vi "Stop Module Event.vi"(8 "error in (no error)":errorcluster, 11 "Action":enum16{"Create", "Get", "Destroy"}(ring)=enum."Destroy") -> (0 "error out":errorcluster, 3 "Stop Module":refnum<user-event>)   [LabVIEW 2018]
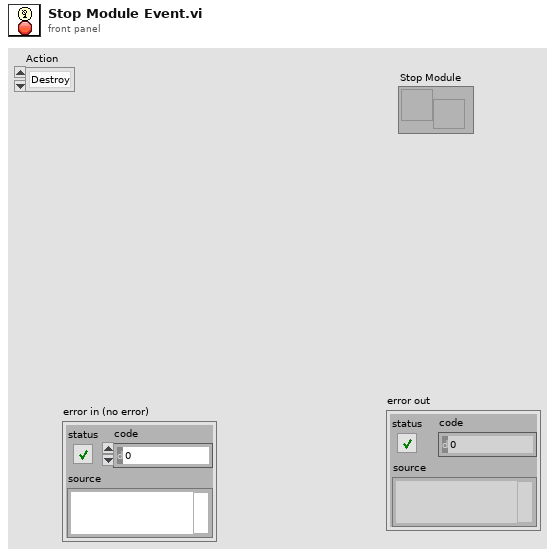
[diagram p1: front panel]
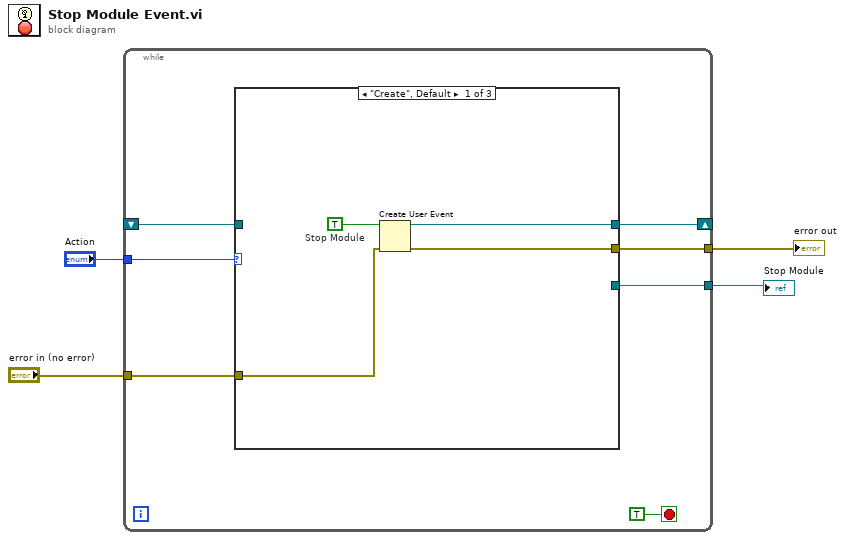
[diagram p0: block diagram]
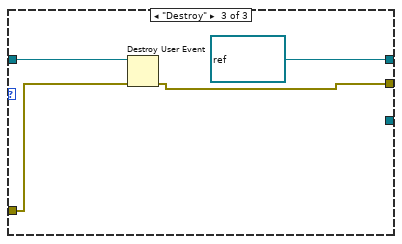
[diagram p3: hidden frame]
diagram:
  n1 = while {
    tunnel: "Action" -> [w10]
    shift-right: [w9] -> _
    shift-left: _ -> [w8]
    tunnel: "error in (no error)" -> [w7]
    tunnel: [w6] -> w2
    tunnel: [w5] -> w1
    stop <- TRUE stop-if-true
    n2 = case shown="\"Create\", Default" w10 {
      tunnel: [w14 w16 refnum<user-event> refnum ("Stop Module")] -> w9
      tunnel: w8 -> [_ w16 w21]
      tunnel: w7 -> [w13 w17 w18]
      tunnel: [w12 w17 w19] -> w6
      tunnel: [_ w16 _] -> w5
      frame "Create", Default {
        w15 = TRUE  # Stop Module
        n3 = Create User Event(user event datatype=w15, error in=w13) -> (user event=w14:refnum<user-event>, error out=w12:errorcluster)
      }
      frame "Get" {
      }
      frame "Destroy" {
        n4 = Destroy User Event(user event=w21, error in=w18) -> (error out=w19:errorcluster)
      }
    }
  }
  "error out" <- w2
  "Stop Module" <- w1
